vi "mode_sensitivity.vi"(0 "reference":refnum<class "OSA200.lvclass">, 2 "sensitivity":u16=3, 5 "error in (no error)":errorcluster, 7 "ctrl ref":refnum<vi>, 9 "read/write":enum16{"read", "write"}(ring)) -> (14 "duplicate reference":refnum<class "OSA200.lvclass">, 16 "sensitivity out":u16=3, 19 "error out":errorcluster)   [LabVIEW 2010, in "OSA200.lvclass"]
doc: "Sensitivity affect settable gain range, (sensitivity high: gain range = 0-15, and sens low: 0 - 11), and sampling intervall, (nr of samples per reference laser period, sens high: 32, low: 16). Sensitivity high recommended for low power sources or for high performance wavemeter resolution. The update rate, (interferogram read), is lower in high sensitivity mode."
uses:
  OSA200.lvclass
  OSA.lvclass
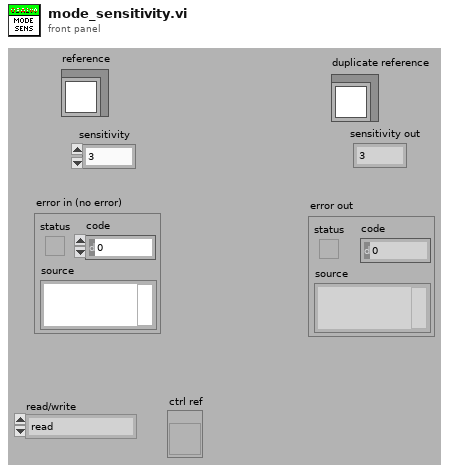
[diagram p1: front panel]
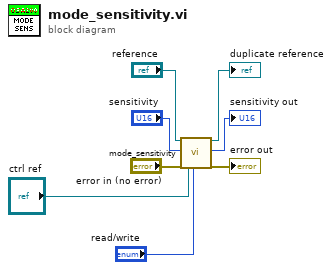
[diagram p0: block diagram]
diagram:
  n1 = call-parent "mode_sensitivity.vi"("reference"="reference", "sensitivity"="sensitivity", "error in (no error)"="error in (no error)", "ctrl ref"="ctrl ref", "read/write"="read/write") -> ("duplicate reference"=→"duplicate reference":refnum<class "OSA200.lvclass">, "sensitivity out"=→"sensitivity out":u16, "error out"=→"error out":errorcluster)  [unwired: 12 in]
